vi "Destroy User Events.vi"(8 "error in":errorcluster, 11 "VF Device Selection in":refnum<class "VF Device Selection.lvclass">) -> (0 "error out":errorcluster, 3 "VF Device Selection out":refnum<class "VF Device Selection.lvclass">)   [LabVIEW 2018, in "VF Device Selection Actor.lvlib" / "VF Device Selection.lvclass"]
uses:
  VF Device Selection.lvclass
  VF Device Selection.lvclass/VF Device Selection.ctl
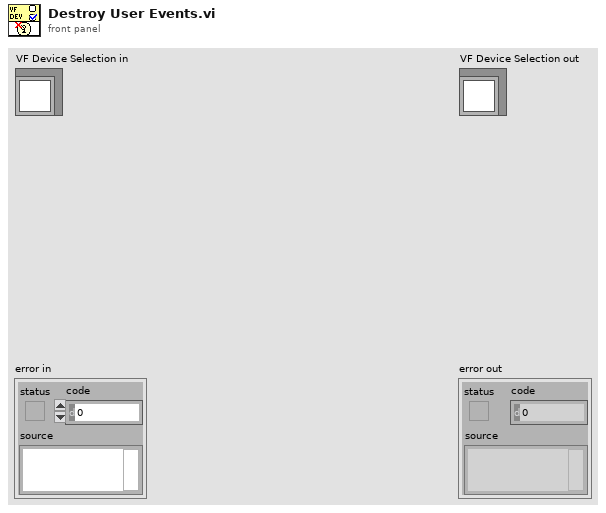
[diagram p1: front panel]
types:
  T1 = typedef "VF Device Selection Actor.lvlib/VF Device Selection.lvclass/VF Device Selection User Events.ctl" = cluster{"ItemNames":refnum<user-event>, "stop":refnum<user-event>}
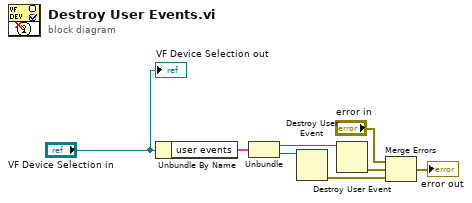
[diagram p0: block diagram]
diagram:
  n1 = Unbundle By Name("VF Device Selection in") -> ("user events"=w6:T1)
  n2 = Unbundle(w6) -> ("ItemNames"=w4:refnum<user-event>, "stop"=w5:refnum<user-event>)
  n3 = Destroy User Event(user event=w5) -> (error out=w1:errorcluster)  [unwired: 1 in]
  n4 = Destroy User Event(user event=w4) -> (error out=w2:errorcluster)  [unwired: 1 in]
  n5 = Merge Errors("error in", w2, w1) -> (→"error out":errorcluster)
  "VF Device Selection out" <- "VF Device Selection in"
